vi "Laser_Closing.vi"(0 "Error In":errorcluster) -> ()   [LabVIEW 2016]
uses:
  Utility/Global_Laser.vi
  Utility/Global Constants.vi
  Program Files (x86)/OPOTEK_DLL/OPOTEK.dll
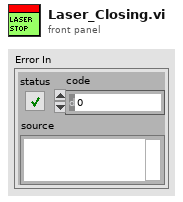
[diagram p1: front panel]
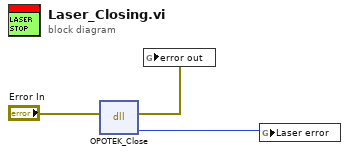
[diagram p0: block diagram]
diagram:
  n1 = dll-call lib="C:/Program Files (x86)/OPOTEK_DLL/OPOTEK.dll" fn="OPOTEK_Close"(error in="Error In") -> (error out=w2:errorcluster, "error_Code"=w1:i32)  [unwired: 4 in, 1 out]
  n2 = global write "Global Constants.vi" "error out"(w2) -> ()
  n3 = global write "Global_Laser.vi" "Laser error"(w1) -> ()
